vi "LV2_2.vi"() -> ()   [LabVIEW 2011]
uses:
  <vilib>/imath/engines/lvmath2/RunTimeEngine/ErrorHandling/NIMS_Finalize Error.vi
  <vilib>/imath/engines/lvmath2/RunTimeEngine/NodeEndStatement/NIMS_NodeEndStatement_Output.vi
  <instcachedir>/0/NIMS_NodeEndStatement_Output_53EC0D466D134D7ABD903AC30B43404B.lvgen/NIMS_NodeEndStatement_Output_53EC0D466D134D7ABD903AC30B43404B_000.vi
  <instcachedir>/0/NIMS_NodeEndStatement_Output_53EC0D466D134D7ABD903AC30B43404B.lvgen/NIMS_NodeEndStatement_Output_53EC0D466D134D7ABD903AC30B43404B_005.vi
  <vilib>/imath/engines/lvmath2/RunTimeEngine/BuiltInFunctions/linramp/NIMS_linramp.vi
  <vilib>/imath/engines/lvmath2/RunTimeEngine/ArithmeticOperatorToken/NIMS_ArithmeticOperator_plus.vi
  <instcachedir>/0/NIMS_ArithmeticOperator_plus_1E95F7DAB906458CBECCADBE8E6FD739.lvgen/NIMS_ArithmeticOperator_plus_1E95F7DAB906458CBECCADBE8E6FD739_001.vi
  <vilib>/imathl/engines/lvmath/Functions/Error Handling/Create Error.vi
  <instcachedir>/0/NIMS_NodeEndStatement_Output_53EC0D466D134D7ABD903AC30B43404B.lvgen/NIMS_NodeEndStatement_Output_53EC0D466D134D7ABD903AC30B43404B_001.vi
  <vilib>/imath/engines/lvmath2/RunTimeEngine/BuiltInFunctions/round/NIMS_round(DBL-S).vi
  <vilib>/imath/engines/lvmath2/RunTimeEngine/BuiltInFunctions/zeros/NIMS_V=zeros(I32,I32).vi
  <vilib>/imath/engines/lvmath2/RunTimeEngine/RangeToken/NIMS_Range.vi
  <instcachedir>/0/NIMS_Range_0B7635FB69F84E19AA68E7FF959DF37C.lvgen/NIMS_Range_0B7635FB69F84E19AA68E7FF959DF37C_001.vi
  <vilib>/imath/engines/lvmath2/RunTimeEngine/VariableToken/Read/NIMS_Get Elements - RV(_) - Check(_).vi
  <instcachedir>/0/NIMS_Get Elements - RV(_) - Check(_)_95E78A4FFA0646428F3543E57837F638.lvgen/NIMS_Get Elements - RV(_) - Check(_)_95E78A4FFA0646428F3543E57837F638_000.vi
  <vilib>/imath/engines/lvmath2/RunTimeEngine/ErrorHandling/NIMS_Create Error From Enums.vi
  <vilib>/imath/engines/lvmath2/RunTimeEngine/BuiltInFunctions/polyval/NIMS_polyval(GV,GM).vi
  <instcachedir>/0/NIMS_polyval(GV,GM)_E12556DC54744E0C81968744501C4F35.lvgen/NIMS_polyval(GV,GM)_E12556DC54744E0C81968744501C4F35_002.vi
  <vilib>/imath/engines/lvmath2/RunTimeEngine/BuiltInFunctions/angle/NIMS_angle.vi
  <instcachedir>/0/NIMS_angle_6DDAE2BD99E0421EB990B6436E94D88F.lvgen/NIMS_angle_6DDAE2BD99E0421EB990B6436E94D88F_002.vi
  <vilib>/imath/engines/lvmath2/RunTimeEngine/BuiltInFunctions/abs/NIMS_abs(signed).vi
  <instcachedir>/0/NIMS_abs(signed)_C4FCB8E6058B49B797C7C8D53CA5F6EC.lvgen/NIMS_abs(signed)_C4FCB8E6058B49B797C7C8D53CA5F6EC_002.vi
panel:
  in  "stop":bool
  out "Car Response":cluster{"t":dbl[], "Y":dbl[]}[](graph)=[{"t"=array[1000 elements], "Y"=array[1000 elements]}, {"t"=[0.0, 0.5], "Y"=[0.6561797752808989, 0.6561797752808989]}]
  in  "spring constant (N/m)":dbl(slide)=88317.75700934579 scale=50000.0..150000.0
  in  "mass (kg)":dbl(slide)=1228.9719626168223 scale=500.0..1500.0
  in  "damping (Ns/m)":dbl(slide)=8785.046728971962 scale=5000.0..20000.0
  in  "Shape":enum32{"Curb", "Pothole", "Wavy pavement"}(tab)
  in  "curb amplitude (cm)":dbl(slide)=0.6561797752808989 scale=0.1..10.0
  in  "speed (m/s)":dbl(knob)=2.006374146470188 scale=2.0..10.0
  in  "width (m)":dbl(slide)=0.1 scale=0.1..1.0
  in  "depth (cm)":dbl(slide)=0.1 scale=0.1..10.0
  in  "amplitude (cm)":dbl(slide)=1.9353932584269664 scale=0.1..10.0
  in  "period (s)":dbl(slide)=0.18595505617977529 scale=0.1..1.0
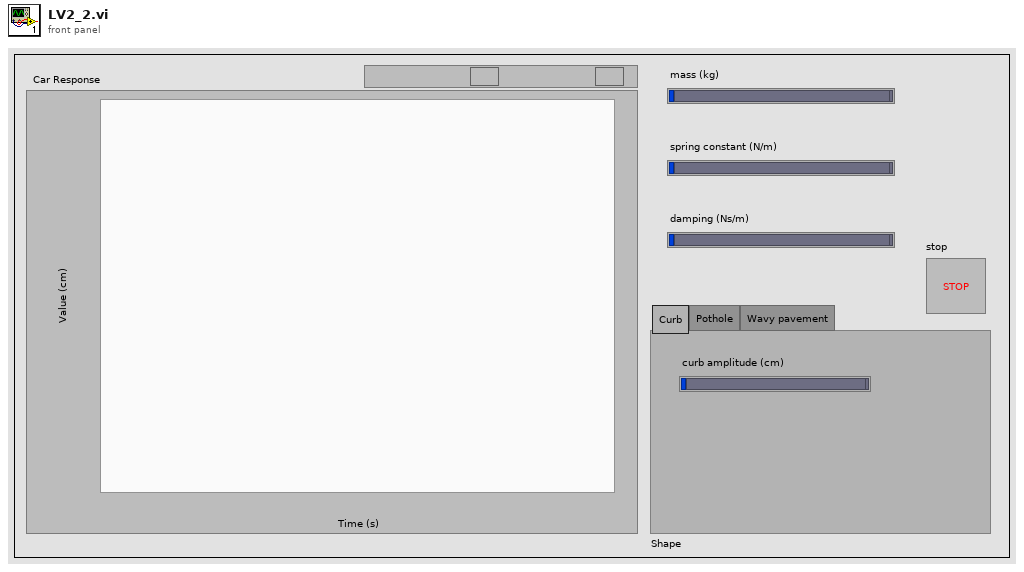
[diagram p1: front panel]
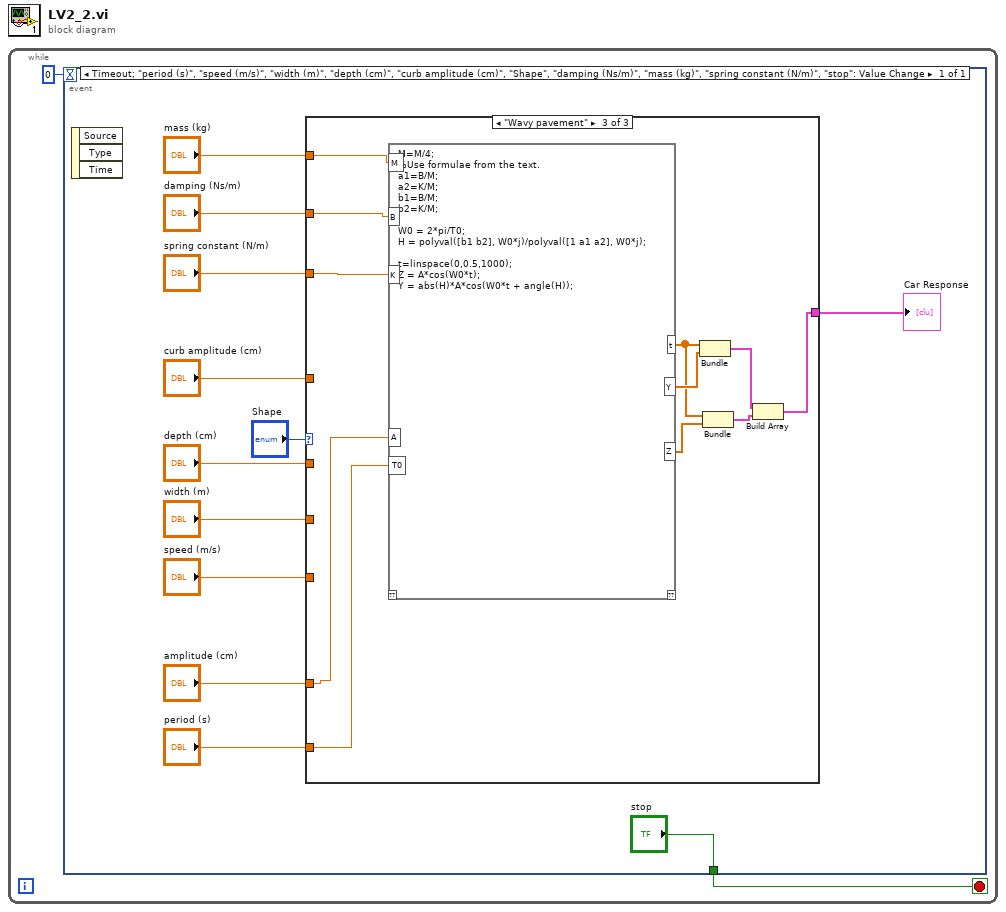
[diagram p0: block diagram]
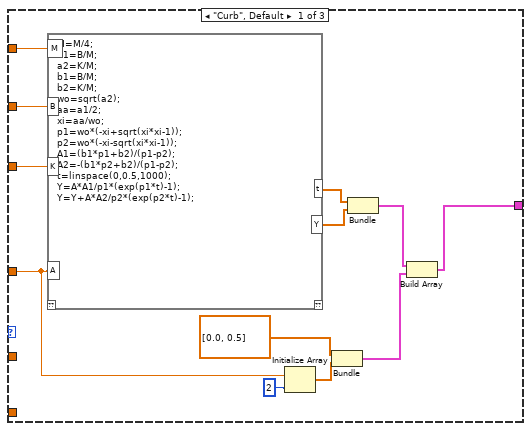
[diagram p2: hidden frame]
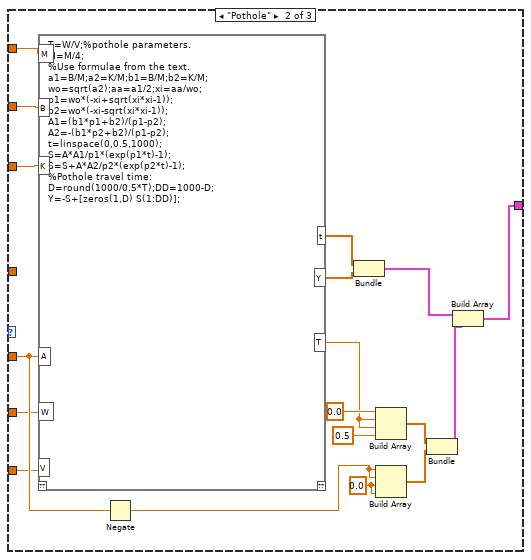
[diagram p3: hidden frame]
diagram:
  n1 = while {
    stop <- w2 stop-if-true
    n2 = event shown="[0] Timeout;  \"period (s)\", \"speed (m/s)\", \"width (m)\", \"depth (cm)\", \"curb amplitude (cm)\", \"Shape\", \"damping (Ns/m)\", \"mass (kg)\", \"spring constant (N/m)\", \"stop\": Value Change" {
      selector: _ -> [_]
      dyn-events: _ -> [_]
      timeout: 0 -> [_]
      tunnel: ["stop"] -> w2
      event Timeout; "period (s)", "speed (m/s)", "width (m)", "depth (cm)", "curb amplitude (cm)", "Shape", "damping (Ns/m)", "mass (kg)", "spring constant (N/m)", "stop": Value Change {
        n3 = event-data() -> ()  [unwired: 1 in, 3 out]
        n4 = case shown="\"Wavy pavement\"" "Shape" {
          tunnel: "mass (kg)" -> [w26 w219 w464]
          tunnel: "damping (Ns/m)" -> [w22 w204 w463]
          tunnel: "spring constant (N/m)" -> [w23 w205 w462]
          tunnel: "curb amplitude (cm)" -> [w21 _ _]
          tunnel: "depth (cm)" -> [_ w212 _]
          tunnel: "width (m)" -> [_ w203 _]
          tunnel: "amplitude (cm)" -> [_ _ w461]
          tunnel: "period (s)" -> [_ _ w460]
          tunnel: "speed (m/s)" -> [_ w202 _]
          tunnel: [w16 w206 w455] -> w3
          frame "Curb", Default {
            n5 = mathscript code="M=M/4;\na1=B/M;\na2=K/M;\nb1=B/M;\nb2=K/M;\nwo=sqrt(a2);\naa=a1/2;\nxi=aa/wo;\np1=wo*(-xi+sqrt(xi*xi-1));\np2=wo*(-xi-sqrt(xi*xi-1));\nA1=(b1*p1+b2)/(p1-p2);\nA2=-(b1*p2+b2)/(p1-p2);\nt=linspace(0,0.5,1000);\nY=A*A1/p1*(exp(p1*t)-1);\nY=Y+A*A2/p2*(exp(p2*t)-1);"("A"=w21, "M"=w26, "K"=w23, "B"=w22) -> ("t"=w25:dbl[], "Y"=w24:cdb[])  [unwired: 1 in, 1 out]
            n6 = Initialize Array(w21, 2 ("dimension size")) -> (w19:dbl[])
            n7 = Bundle(dbl[] [0.0, 0.5], w19) -> (w17:cluster{dbl[], dbl[]})  [unwired: 1 in]
            n8 = Bundle("t"=w25, "Y"=w24) -> (w18:cluster{"t":dbl[], "Y":cdb[]})  [unwired: 1 in]
            n9 = Build Array(w18, w17) -> (w16:cluster{"t":dbl[], "Y":cdb[]}[])
          }
          frame "Pothole" {
            w213 = 0.0 ("element")
            n10 = mathscript code="T=W/V;%pothole parameters.\nM=M/4;\n%Use formulae from the text.\na1=B/M;a2=K/M;b1=B/M;b2=K/M;\nwo=sqrt(a2);aa=a1/2;xi=aa/wo;\np1=wo*(-xi+sqrt(xi*xi-1));\np2=wo*(-xi-sqrt(xi*xi-1));\nA1=(b1*p1+b2)/(p1-p2);\nA2=-(b1*p2+b2)/(p1-p2);\nt=linspace(0,0.5,1000);\nS=A*A1/p1*(exp(p1*t)-1);\nS=S+A*A2/p2*(exp(p2*t)-1);\n%Pothole travel time:\nD=round(1000/0.5*T);DD=1000-D;\nY=-S+[zeros(1,D) S(1:DD)];"("A"=w212, "W"=w203, "V"=w202, "M"=w219, "K"=w205, "B"=w204) -> ("t"=w218:dbl[], "Y"=w217:cdb[], "T"=w215:dbl)  [unwired: 1 in, 1 out]
            n11 = Negate(x=w212) -> (-x=w211:dbl)
            n12 = Bundle("t"=w218, "Y"=w217) -> (w208:cluster{"t":dbl[], "Y":cdb[]})  [unwired: 1 in]
            n13 = Build Array(0.0 ("element"), w215, w215, 0.5 ("element")) -> (w210:dbl[])
            n14 = Build Array(w211, w211, w213, w213) -> (w209:dbl[])
            n15 = Bundle(w210, w209) -> (w207:cluster{dbl[], dbl[]})  [unwired: 1 in]
            n16 = Build Array(w208, w207) -> (w206:cluster{"t":dbl[], "Y":cdb[]}[])
          }
          frame "Wavy pavement" {
            n17 = mathscript code="M=M/4;\n%Use formulae from the text.\na1=B/M;\na2=K/M;\nb1=B/M;\nb2=K/M;\n\nW0 = 2*pi/T0;\nH = polyval([b1 b2], W0*j)/polyval([1 a1 a2], W0*j);\n\nt=linspace(0,0.5,1000);\nZ = A*cos(W0*t);\nY = abs(H)*A*cos(W0*t + angle(H));"("T0"=w460, "A"=w461, "M"=w464, "K"=w462, "B"=w463) -> ("t"=w458:dbl[], "Y"=w459:dbl[], "Z"=w457:dbl[])  [unwired: 1 in, 1 out]
            n18 = Bundle("t"=w458, "Y"=w459) -> (w456:cluster{"t":dbl[], "Y":dbl[]})  [unwired: 1 in]
            n19 = Bundle("t"=w458, "Z"=w457) -> (w454:cluster{"t":dbl[], "Z":dbl[]})  [unwired: 1 in]
            n20 = Build Array(w456, w454) -> (w455:cluster{"t":dbl[], "Z":dbl[]}[])
          }
        }
        "Car Response" <- w3
      }
    }
  }
